vi "Logging Cache.vi"(4 "error in (no error)":errorcluster, 5 "Variable":T2, 6 "Mode":T3(ring), 7 "LoggingDevRef":T1) -> (0 "error out":errorcluster, 1 "Out":T2[](array[typedef]), 3 "LoggingDevRef":T1)   [LabVIEW 2012, in "femtoRoboLib.lvlib"]
uses:
  femtoRoboLib.lvlib
  Log Entry - Converted.ctl
  LoggingDevRef.ctl
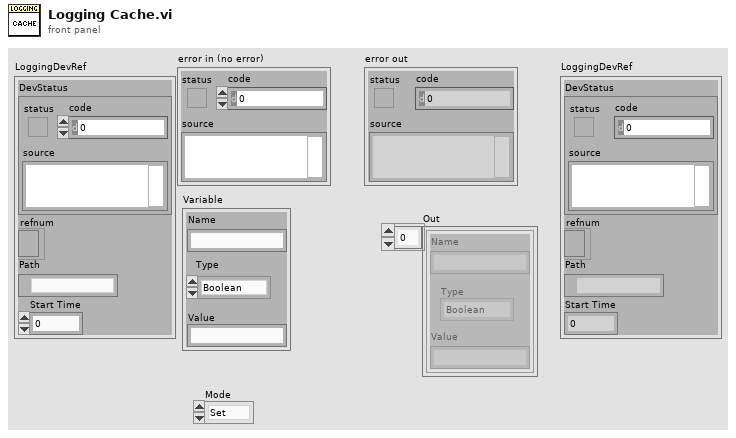
[diagram p1: front panel]
types:
  T1 = typedef "femtoRoboLib.lvlib/LoggingDevRef.ctl" = cluster{"DevStatus":errorcluster, "refnum":refnum<file>, "Path":path, "Start Time":u32}
  T2 = typedef "femtoRoboLib.lvlib/Log Entry - Converted.ctl" = cluster{"Name":string, "Type":enum16{"Boolean", "Numeric", "String", "Boolean Array", "Numeric Array", "String Array"}, "Value":string}
  T3 = enum16{"Set", "Get Unsaved", "Get Unsaved and Clear", "Get All"}
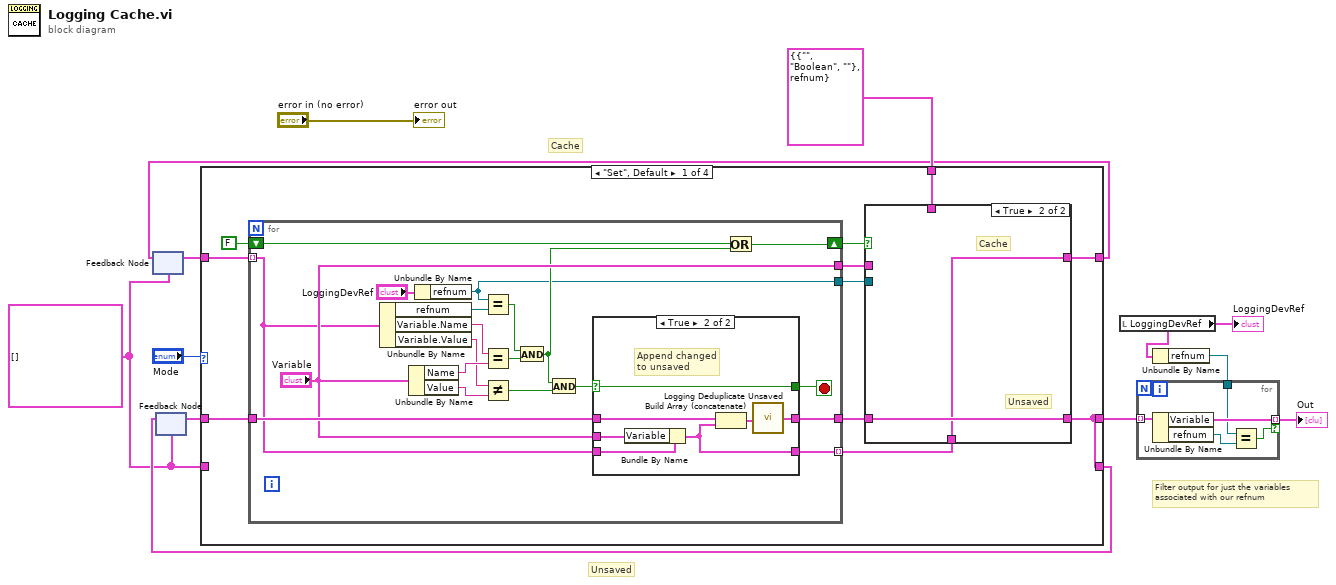
[diagram p0: block diagram]
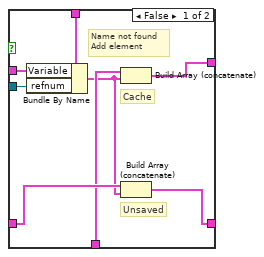
[diagram p2: hidden frame]
diagram:
  w8 = cluster{"Variable":T2, "refnum":refnum<file>}[] [] ("Cache")
  # "Cache"
  # "Filter output for just the variables\nassociated with our refnum"
  # "Unsaved"
  n1 = feedback #1(w8) -> (w12:cluster{"Variable":T2, "refnum":refnum<file>}[])
  n2 = feedback #2(w8) -> (w11:cluster{"Variable":T2, "refnum":refnum<file>}[])
  n3 = case shown="\"Set\", Default" "Mode" {
    tunnel: w12 -> [w15 w64 w66 w69]
    tunnel: w11 -> [w23 w65 w67 w70]
    tunnel: [w18 w65 w67 w69] -> w5
    tunnel: w8 -> [_ _ w68 _]
    tunnel: [w18 w65 w68 w70] -> w9
    tunnel: cluster{"Variable":T2, "refnum":refnum<file>} {"Variable"={"Name"="", "Type"=enum."Boolean", "Value"=""}, "refnum"=refnum} ("Cache Entry") -> [w16 _ _ _]
    tunnel: [w14 w64 w66 w69] -> w6
    frame "Set", Default {
      n4 = for {
        tunnel: w15 -> [w37] mode=indexing
        tunnel: [w48] -> w19
        tunnel: w23 -> [w49]
        shift-right: [w46] -> w20
        shift-left: FALSE -> [w47]
        tunnel: ["Variable"] -> w21
        tunnel: [w36] -> w17
        tunnel: [w35] -> w13 mode=indexing
        stop <- w34 stop-if-true
        n5 = Unbundle By Name(w37) -> ("refnum"=w43:refnum<file>, "Variable.Name"=w53:string, "Variable.Value"=w51:string)
        n6 = Unbundle By Name("Variable") -> ("Name"=w52:string, "Value"=w50:string)
        n7 = Unbundle By Name("LoggingDevRef") -> ("refnum"=w36:refnum<file>)
        n8 = Equal?(x=w36, y=w43) -> (x = y?=w42:bool)
        n9 = Equal?(x=w53, y=w52) -> (x = y?=w41:bool)
        n10 = Not Equal?(x=w51, y=w50) -> (x != y?=w38:bool)
        n11 = And(x=w42, y=w41) -> (x .and. y?=w39:bool)
        n12 = And(x=w39, y=w38) -> (x .and. y?=w40:bool)
        n13 = case shown="True" w40 {
          selector: w40 -> [w54 w59]
          tunnel: "Variable" -> [_ w62]
          tunnel: [w56 w57] -> w48
          tunnel: w49 -> [w56 w63]
          tunnel: w37 -> [w55 w61]
          tunnel: [w55 w60] -> w35
          tunnel: [w54 w59] -> w34
          frame False {
          }
          frame True {
            # "Append changed\nto unsaved"
            n14 = Bundle By Name(cluster=w61, "Variable"=w62) -> (w60:cluster{"Variable":T2, "refnum":refnum<file>})
            n15 = Build Array (concatenate)(w63, w60) -> (w58:cluster{"Variable":T2, "refnum":refnum<file>}[])
            n16 = call "Logging Deduplicate Unsaved.vi"("Input"=w58) -> ("Output"=w57:cluster{"Variable":T2, "refnum":refnum<file>}[])
          }
        }
        n17 = Or(x=w47, y=w39) -> (x .or. y?=w46:bool)
      }
      n18 = case shown="True" w20 {
        tunnel: w21 -> [w28 _]
        tunnel: w19 -> [w31 w33]
        tunnel: [w30 w33] -> w18
        tunnel: w17 -> [w27 _]
        tunnel: w16 -> [w29 _]
        tunnel: [w26 w32] -> w14
        tunnel: w13 -> [w25 w32]
        frame False {
          # "Cache"
          # "Unsaved"
          # "Name not found\nAdd element"
          n19 = Bundle By Name(cluster=w29, "Variable"=w28, "refnum"=w27) -> (w24:cluster{"Variable":T2, "refnum":refnum<file>})
          n20 = Build Array (concatenate)(w25, w24) -> (w26:cluster{"Variable":T2, "refnum":refnum<file>}[])
          n21 = Build Array (concatenate)(w31, w24) -> (w30:cluster{"Variable":T2, "refnum":refnum<file>}[])
        }
        frame True {
          # "Cache"
          # "Unsaved"
        }
      }
    }
    frame "Get Unsaved" {
      # "Cache = Cache"
      # "Unsaved = Unsaved"
      # "Output = Unsaved"
    }
    frame "Get Unsaved and Clear" {
      # "Cache = Cache"
      # "Output = Unsaved"
      # "Unsaved = Empty"
    }
    frame "Get All" {
      # "Unsaved = Unsaved"
      # "Cache = Cache"
      # "Output = Cache"
    }
  }
  n22 = feedback-in #1(w6) -> ()
  n23 = feedback-in #2(w9) -> ()
  n24 = local read "LoggingDevRef"() -> (w2:T1)
  "LoggingDevRef" <- w2
  n25 = Unbundle By Name(w2) -> ("refnum"=w3:refnum<file>)
  n26 = for {
    tunnel: w5 -> [w75] mode=indexing
    tunnel: [w74] -> w4 mode=indexing if=w73
    tunnel: w3 -> [w72]
    n27 = Unbundle By Name(w75) -> ("Variable"=w74:T2, "refnum"=w71:refnum<file>)
    n28 = Equal?(x=w72, y=w71) -> (x = y?=w73:bool)
  }
  "Out" <- w4
  "error out" <- "error in (no error)"
